vi "Dispose.vi"(0 "Display State In":T1, 9 "Container State":T2, 11 "error in (no error)":errorcluster) -> (4 "Display State Out":T1, 15 "error out":errorcluster)   [LabVIEW 2020, in "WebView2 Control.xctl"]
uses:
  WebView2 Control.xctl
  <vilib>/_xctls/Container State.ctl
  State.ctl
  Webview2 Lib/WebView2 Control Object/WebView2 Control.lvclass
  <vilib>/_xctls/XControlSupport.lvlib
panel:
  # "Add Controls & Indicators that form the parameters of the method here. Hook them to the connector pane. Do not delete the controls & indicators that are already hooked to the connector pane.\n \nTo setup the parameters  for this method, right click on this item in the Project Tree & select \"Configure Method...\"."
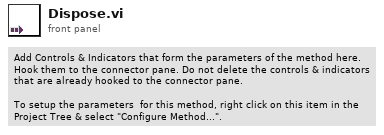
[diagram p1: front panel]
types:
  T1 = typedef "WebView2 Control.xctl/State.ctl" = cluster{"Control Object Ref":refnum<data-value>}
  T2 = typedef "XControlSupport.lvlib/Container State.ctl" = cluster{"Indicator?":bool, "Run Mode?":bool, " Refnum":refnum<vi>}
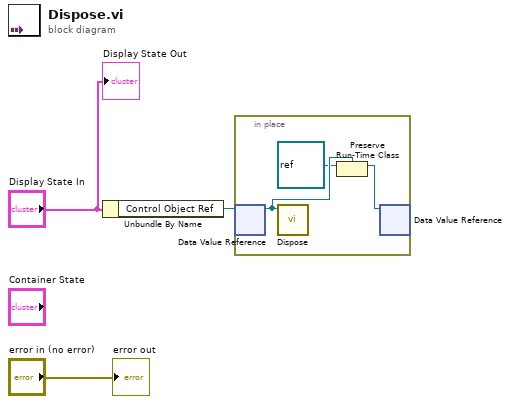
[diagram p0: block diagram]
diagram:
  n1 = Unbundle By Name("Display State In") -> ("Control Object Ref"=w1:refnum<data-value>)
  n2 = in-place {
    n3 = in-place-dvr #1(w1) -> (w6:refnum<class "WebView2 Control.lvclass">)  [unwired: 1 out]
    n4 = call "Dispose.vi"("WebView2 Control in"=w6) -> ()  [unwired: 10 in, 1 out]
    n5 = Preserve Run-Time Class(object in=refnum<class> refnum, 2:w6) -> (object out=w5:refnum<class "WebView2 Control.lvclass">)  [unwired: 1 in, 1 out]
    n6 = in-place-dvr #1(w5) -> ()  [unwired: 2 out]
  }
  "Display State Out" <- "Display State In"
  "error out" <- "error in (no error)"
